vi "WSVCAP SHL Host TL I2C Configure.vi"(0 "I2C_Slave Address":u8=20, 9 "Clock Rate (Hz)":dbl=50000.0, 11 "error in":errorcluster, 13 "Log (T)":bool=TRUE, 14 "FPGA":T1) -> (6 "Actual Rate (Hz)":dbl, 15 "error out":errorcluster)   [LabVIEW 2017]
uses:
  Type Defs/WSVCAP SHL FPGA Enum.ctl
  Type Defs/WSVCAP SHL Function Enum.ctl
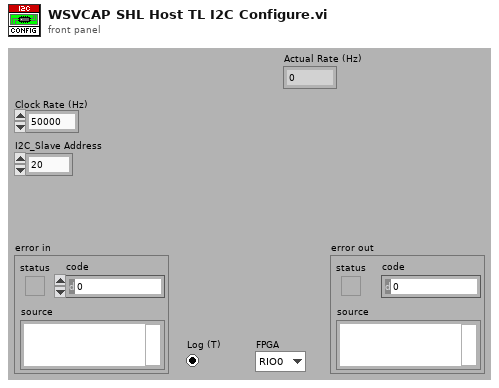
[diagram p1: front panel]
types:
  T1 = typedef "WSVCAP SHL FPGA Enum.ctl" = enum16{"RIO0", "RIO1"}
  T2 = typedef "WSVCAP SHL Function Enum.ctl" = enum16{"Initialize", "Configure I2C", "Configure SRL", "Write I2C", "Read I2C", "Write SRL", "Start SRL Cycle", "Stop SRL Cycle", "Get Status", "Close"}
  T3 = typedef "WSVCAP SHL Core System Cluster.ctl" = cluster{"Settings":T4, "FPGA Resource":tag, "Online":bool, "I2C Wait Ticks":u32, "SRL Wait Ticks":u32, "FPGA VI Reference (FPGA Mode)":T5, "FPGA VI Reference (Sim Mode)":refnum<vi>}
  T4 = typedef "WSVCAP SHL I2C Settings Cluster.ctl" = cluster{"I2C Slave Address":u8, "I2C Clock Rate (Hz)":dbl, "SRL Clock Rate (Hz)":dbl, "Simulate FPGA":bool, "C1 Cap DAC Default":u8, "C2 Cap DAC Default":u8, "C3 Cap DAC Default":u8, "C4 Cap DAC Default":u8, "DAC Out Vref (V)":dbl}
  T5 = typedef "WSVCAP SHL FPGA Ref.ctl" = refnum<k20>
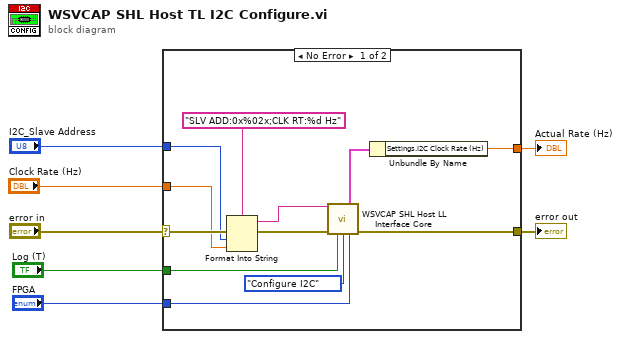
[diagram p0: block diagram]
diagram:
  n1 = case shown="No Error" "error in" {
    selector: "error in" -> [w17 w20]
    tunnel: [w19 w20] -> w6
    tunnel: "Clock Rate (Hz)" -> [w15 _]
    tunnel: "I2C_Slave Address" -> [w14 _]
    tunnel: [w11 _] -> w3
    tunnel: "Log (T)" -> [w9 _]
    tunnel: "FPGA" -> [w8 _]
    frame No Error {
      n2 = Format Into String(format string="SLV ADD:0x%02x;CLK RT:%d Hz", error in=w17, w14, w15) -> (resulting string=w13:string, error out=w16:errorcluster)  [unwired: 1 in]
      n3 = call "WSVCAP SHL Host LL Interface Core.vi"("Message In"=w13, "error in"=w16, "Log (T)"=w9, "Function"=WSVCAP_SHL_Function_Enum."Configure I2C", "FPGA"=w8) -> ("System"=w12:T3, "error out"=w19:errorcluster)  [unwired: 8 in, 1 out]
      n4 = Unbundle By Name(w12) -> ("Settings.I2C Clock Rate (Hz)"=w11:dbl)
    }
    frame Error {
    }
  }
  "Actual Rate (Hz)" <- w3
  "error out" <- w6
